vi "PASCO_PID.vi"(0 "Delta":dbl(slide) scale=-1.0..1.0, 9 "Integral Reset":bool, 12 "P Gain":dbl=1.0, 13 "I Gain":dbl, 14 "D Gain":dbl) -> (4 "Power Out":dbl, 15 "IsThere":bool)   [LabVIEW 2013]
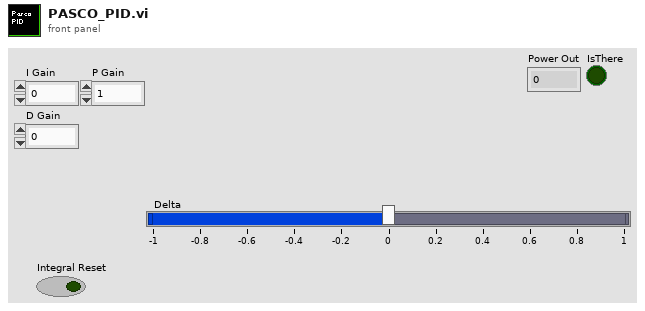
[diagram p1: front panel]
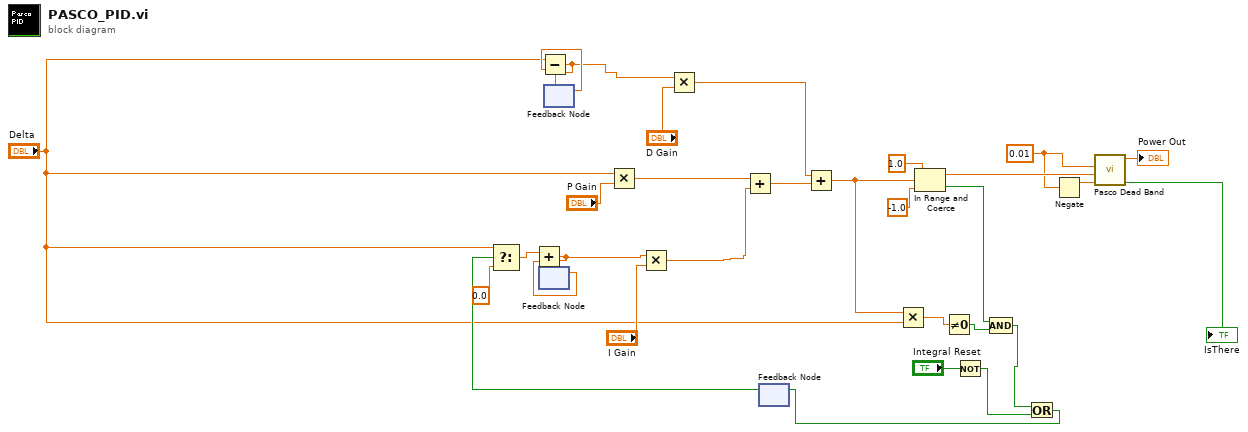
[diagram p0: block diagram]
diagram:
  w16 = 0.01 ("upper limit")
  n1 = feedback #1() -> (w4:dbl)  [unwired: 1 in]
  n2 = feedback #2() -> (w27:dbl)  [unwired: 1 in]
  n3 = Subtract(x="Delta", y=w27) -> (x-y=w5:dbl)
  n4 = feedback-in #2(w5) -> ()
  n5 = Multiply(x="Delta", y="P Gain") -> (x*y=w13:dbl)
  n6 = Multiply(x=w5, y="D Gain") -> (x*y=w6:dbl)
  n7 = feedback #3() -> (w15:bool)  [unwired: 1 in]
  n8 = Select(t="Delta", s=w15, f=0.0) -> (s? t:f=w21:dbl)
  n9 = Add(x=w21, y=w4) -> (x+y=w3:dbl)
  n10 = feedback-in #1(w3) -> ()
  n11 = Multiply(x=w3, y="I Gain") -> (x*y=w7:dbl)
  n12 = Add(x=w13, y=w7) -> (x+y=w20:dbl)
  n13 = Add(x=w6, y=w20) -> (x+y=w19:dbl)
  n14 = Multiply(x=w19, y="Delta") -> (x*y=w25:dbl)
  n15 = In Range and Coerce(upper limit=1.0, x=w19, lower limit=-1.0) -> (coerced(x)=w18:dbl, In Range?=w23:bool)
  n16 = Not Equal To 0?(x=w25) -> (x != 0?=w24:bool)
  n17 = Not(x="Integral Reset") -> (.not. x?=w10:bool)
  n18 = Compound Arithmetic op=AND(w23, w24) -> (w11:bool)
  n19 = Or(x=w11, y=w10) -> (x .or. y?=w9:bool)
  n20 = feedback-in #3(w9) -> ()
  n21 = Negate(x=w16) -> (-x=w17:dbl)
  n22 = call "Pasco Dead Band.vi"("lower limit"=w17, "PWM Power"=w18, "upper limit"=w16) -> ("Integral Reset"=→"IsThere":bool, "PWM Power"=→"Power Out":dbl)  [unwired: 7 in]
